vi "svfa_Build dB Label from Weighting and Ref.vi"(4 "width (-)":i16, 5 "number format":i16(ring) items=["Engineering", "Exponential", "Fractional", "Automatic"], 7 "include reference (T)":bool=TRUE, 8 "error in (no error)":errorcluster, 9 "precision (1)":i16=1, 10 "weighting filter":T1 items=["Linear", "A-weighting", "B-weighting", "C-weighting", "ITU-R 468-4", "Dolby", "CCITT", "C-message", "Wb", "Wc", "Wd", "We", "Wf", "Wh", "Wj", "Wk", "Wm", "AES17 20 kHz lowpass", "AES17 40 kHz lowpass", "AES17 20 kHz highpass", "AES17 40 kHz highpass"], 11 "dB reference [EU]":dbl) -> (0 "error out":errorcluster, 2 "ref label":string, 3 "dB( )":string)   [LabVIEW 2017]
uses:
  <vilib>/addons/_NISVFA/_Shared subVIs/Controls/svc_Weighting Filter Text Ring.ctl
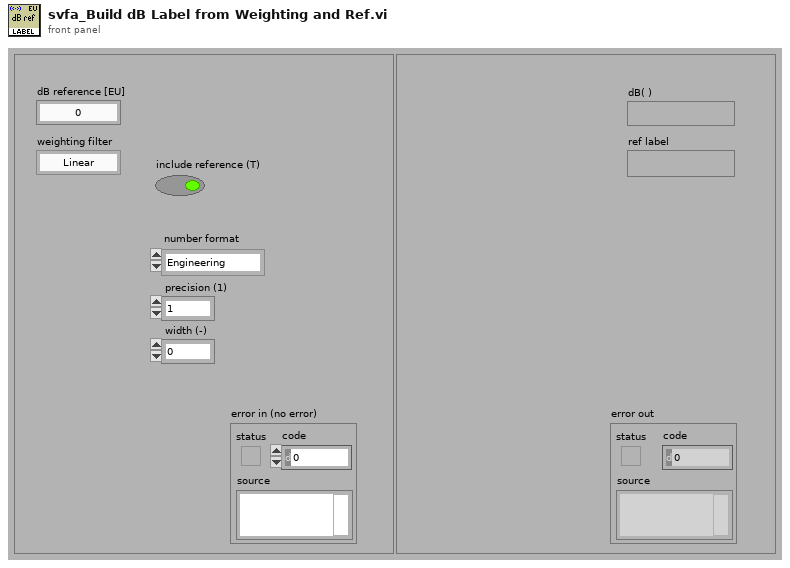
[diagram p1: front panel]
types:
  T1 = typedef "svc_Weighting Filter Text Ring.ctl" = u16
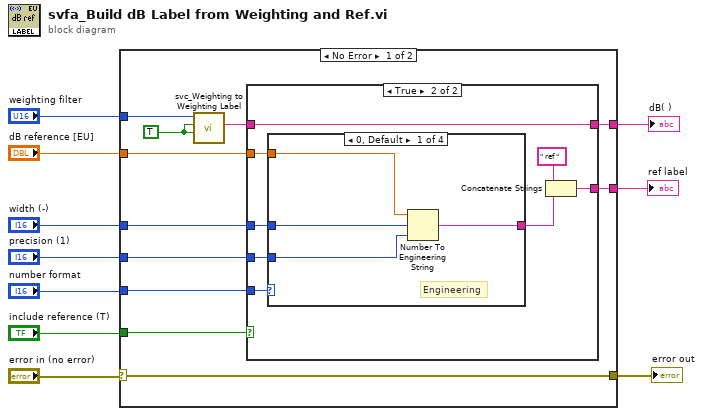
[diagram p0: block diagram]
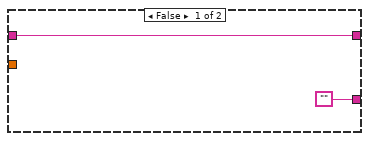
[diagram p2: hidden frame]
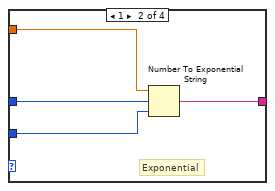
[diagram p3: hidden frame]
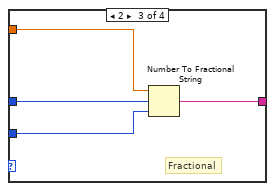
[diagram p4: hidden frame]
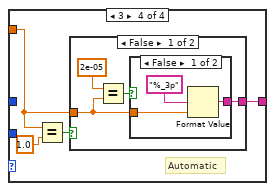
[diagram p5: hidden frame]
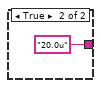
[diagram p6: hidden frame]
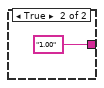
[diagram p7: hidden frame]
diagram:
  n1 = case shown="No Error" "error in (no error)" {
    selector: "error in (no error)" -> [w19 w57]
    tunnel: "include reference (T)" -> [w21 _]
    tunnel: [w20 _] -> w8
    tunnel: [w19 w57] -> w7
    tunnel: "number format" -> [w18 _]
    tunnel: [w17 _] -> w5
    tunnel: "weighting filter" -> [w14 _]
    tunnel: "dB reference [EU]" -> [w13 _]
    tunnel: "precision (1)" -> [w12 _]
    tunnel: "width (-)" -> [w11 _]
    frame No Error {
      w15 = TRUE ("dB On (T)")
      n2 = call <vilib>:"svc_Weighting to Weighting Label.vi"("include weighting if dB On False (T)"=w15, "dB On (T)"=w15, "weighting filter"=w14) -> ("weighting string"=w16:string)  [unwired: 7 in, 1 out]
      n3 = case shown="True" w21 {
        tunnel: ["" ("Empty String Constant") w30] -> w20
        tunnel: w16 -> [w23 w29]
        tunnel: w13 -> [_ w28]
        tunnel: w18 -> [_ w27]
        tunnel: [w23 w29] -> w17
        tunnel: w12 -> [_ w26]
        tunnel: w11 -> [_ w25]
        frame False {
        }
        frame True {
          n4 = case shown="0, Default" w27 {
            tunnel: [w33 w39 w43 w47] -> w24
            tunnel: w25 -> [w34 w38 w42 _]
            tunnel: w26 -> [w35 w37 w41 _]
            tunnel: w28 -> [w32 w36 w40 w46]
            frame 0, Default {
              # "Engineering"
              n5 = Number To Engineering String(2:w35, 3:w34, 4:w32) -> (0:w33:string)  [unwired: 1 in]
            }
            frame 1 {
              # "Exponential"
              n6 = Number To Exponential String(number=w36, precision (6)=w37, 3:w38) -> (E-format string=w39:string)  [unwired: 1 in]
            }
            frame 2 {
              # "Fractional"
              n7 = Number To Fractional String(number=w40, width (-)=w42, precision (6)=w41) -> (F-format string=w43:string)  [unwired: 1 in]
            }
            frame 3 {
              # "Automatic"
              n8 = Equal?(x=w46, y=1.0) -> (x = y?=w44:bool)
              n9 = case shown="False" w44 {
                tunnel: [w51 "1.00" ("format string")] -> w47
                tunnel: w46 -> [w50 _]
                frame False {
                  n10 = Equal?(x=2e-05 ("y"), y=w50) -> (x = y?=w48:bool)
                  n11 = case shown="False" w48 {
                    tunnel: [w53 "20.0u" ("format string")] -> w51
                    tunnel: w50 -> [w52 _]
                    frame False {
                      n12 = Format Value(format string="%_3p", value (0)=w52) -> (output string=w53:string)  [unwired: 1 in]
                    }
                    frame True {
                    }
                  }
                }
                frame True {
                }
              }
            }
          }
          n13 = Concatenate Strings(" ref ", w24) -> (w30:string)
        }
      }
    }
    frame Error {
    }
  }
  "error out" <- w7
  "ref label" <- w8
  "dB( )" <- w5
